vi "Convert Joystick Throttle.vi"(1 "Input":dbl) -> (0 "Output":dbl)   [LabVIEW 2014]
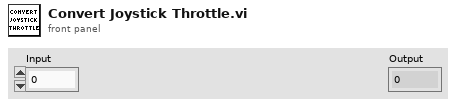
[diagram p1: front panel]
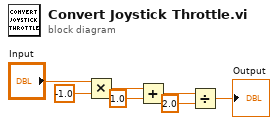
[diagram p0: block diagram]
diagram:
  n1 = Multiply(x="Input", y=-1.0) -> (x*y=w4:dbl)
  n2 = Add(x=w4, y=1.0) -> (x+y=w6:dbl)
  n3 = Divide(x=w6, y=2.0) -> (x/y=→"Output":dbl)
